vi "Write TC Temperature.vi"(8 "error in (no error)":errorcluster, 10 "TC Temperature":waveform(dbl)[](array[waveform]), 11 "DeepU Results in":refnum<class "DeepU Results.lvclass">) -> (0 "error out":errorcluster, 3 "DeepU Results out":refnum<class "DeepU Results.lvclass">)   [LabVIEW 2019, in "Results.lvlib" / "DeepU Results.lvclass"]
uses:
  DeepU Results.lvclass
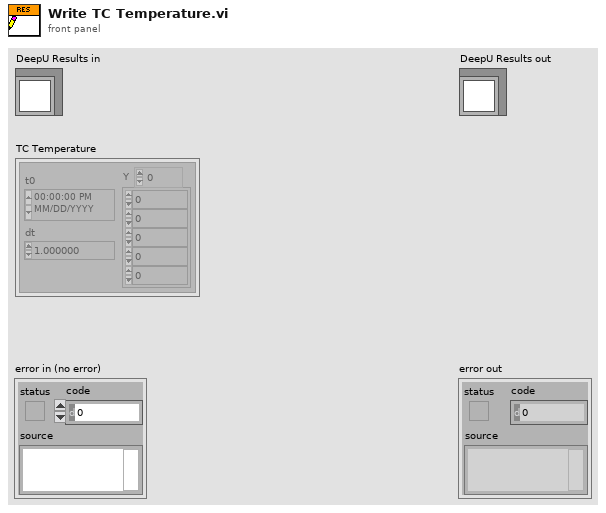
[diagram p1: front panel]
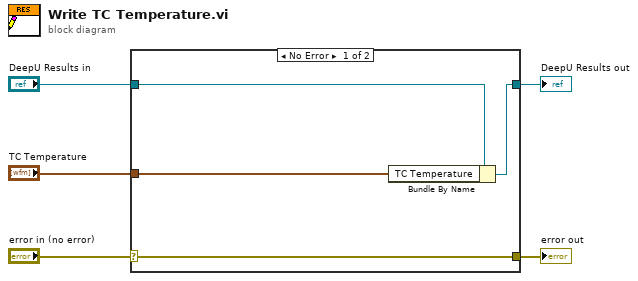
[diagram p0: block diagram]
diagram:
  n1 = case shown="No Error" "error in (no error)" {
    selector: "error in (no error)" -> [w9 w10]
    tunnel: [w9 w10] -> w4
    tunnel: [w7 w11] -> w2
    tunnel: "DeepU Results in" -> [w8 w11]
    tunnel: "TC Temperature" -> [w6 _]
    frame No Error {
      n2 = Bundle By Name(cluster=w8, "TC Temperature"=w6) -> (w7:refnum<class "DeepU Results.lvclass">)
    }
    frame Error {
    }
  }
  "error out" <- w4
  "DeepU Results out" <- w2
